vi "PAQmem_GetPointers.vi"(8 "error in (no error)":errorcluster, 11 "PAQ-memory in":refnum<class "PAQ-memory.lvclass">) -> (0 "error out":errorcluster, 2 "Pointers":cluster{"Pointer":i32, "Carry":i32}, 3 "PAQ-memory out":refnum<class "PAQ-memory.lvclass">)   [LabVIEW 2020, in "PAQ-memory.lvclass"]
doc: "Get memory object pointer and carry value"
uses:
  PAQ-memory.lvclass
  PAQ-memory.lvclass/PAQ-memory.ctl
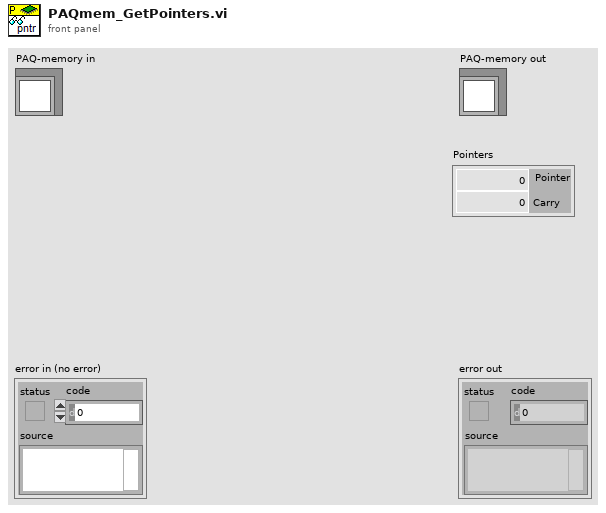
[diagram p1: front panel]
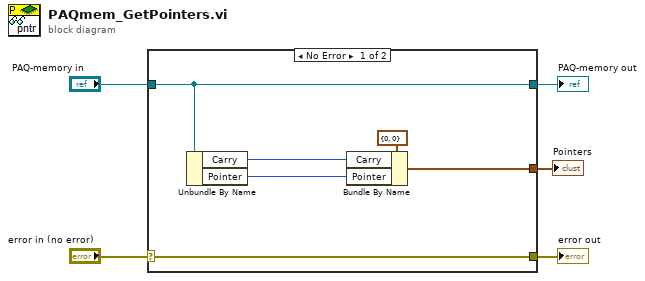
[diagram p0: block diagram]
diagram:
  n1 = case shown="No Error" "error in (no error)" {
    selector: "error in (no error)" -> [w11 w12]
    tunnel: [w11 w12] -> w4
    tunnel: [w10 w13] -> w2
    tunnel: "PAQ-memory in" -> [w10 w13]
    tunnel: [w6 _] -> w1
    frame No Error {
      n2 = Unbundle By Name(w10) -> ("Carry"=w8:i32, "Pointer"=w7:i32)
      n3 = Bundle By Name(cluster=cluster{"Pointer":i32, "Carry":i32} {"Pointer"=0, "Carry"=0} ("Pointers"), "Carry"=w8, "Pointer"=w7) -> (w6:cluster{"Pointer":i32, "Carry":i32})
    }
    frame Error {
    }
  }
  "error out" <- w4
  "PAQ-memory out" <- w2
  "Pointers" <- w1
